vi "均衡解析.vi"(8 "位置":i32, 9 "均衡标记":i32[][](array[numeric]), 11 "均衡引用":refnum<vi>) -> (0 "故障":string[](array[string]), 3 "均衡颜色":u32[](array[colorbox]))   [LabVIEW 2013]
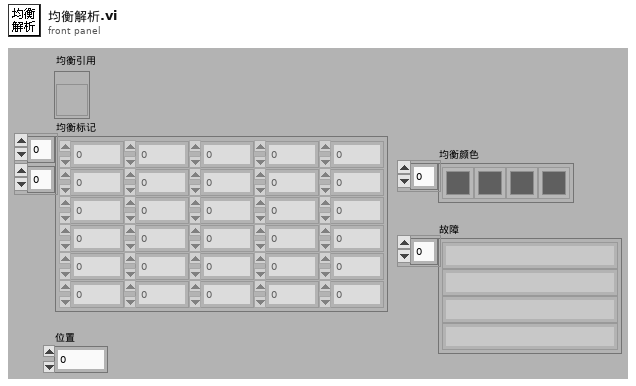
[diagram p1: front panel]
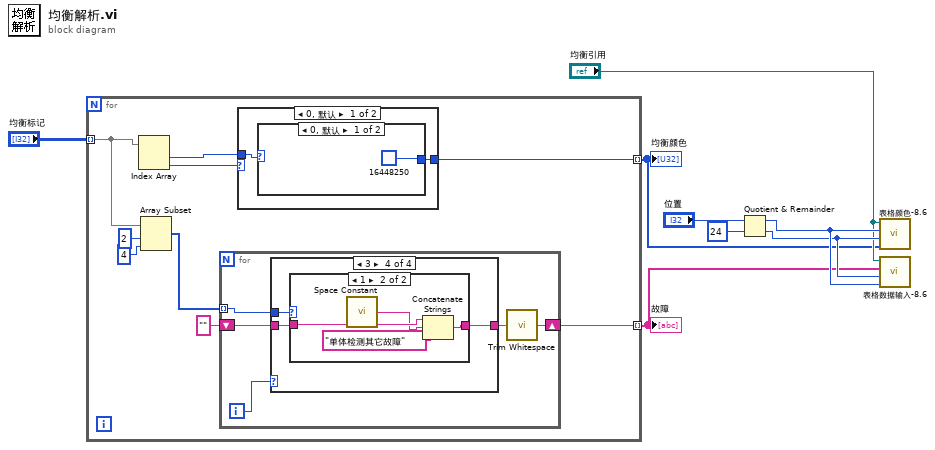
[diagram p0: block diagram]
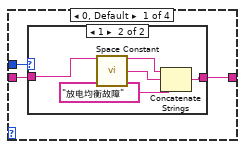
[diagram p2: hidden frame]
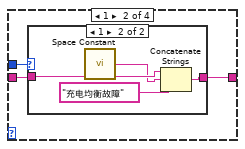
[diagram p4: hidden frame]
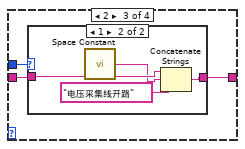
[diagram p6: hidden frame]
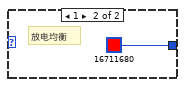
[diagram p9: hidden frame]
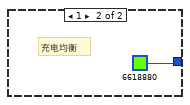
[diagram p10: hidden frame]
diagram:
  n1 = for {
    tunnel: "均衡标记" -> [w14] mode=indexing
    tunnel: [w15] -> w1 mode=indexing
    tunnel: [w9] -> w2 mode=indexing
    n2 = Index Array(array=w14) -> (element #1=w16:i32, element #2=w17:i32)  [unwired: 2 in]
    n3 = Array Subset(array=w14, index=2 ("索引"), length=4 ("长度")) -> (w11:i32[])
    n4 = for {
      tunnel: w11 -> [w22] mode=indexing
      shift-right: [w18] -> w9
      shift-left: "" -> [w20]
      i -> [w19]
      n5 = case shown="3" w19 {
        tunnel: w22 -> [w25 w33 w41 w49]
        tunnel: [w24 w32 w40 w48] -> w21
        tunnel: w20 -> [w23 w31 w39 w47]
        frame 0, Default {
          n6 = case shown="1" w25 {
            tunnel: w23 -> [w26 w28]
            tunnel: [w26 w29] -> w24
            frame 0, Default {
            }
            frame 1 {
              n7 = call <vilib>:"Space Constant.vi"() -> ("String"=w27:string)
              n8 = Concatenate Strings(w28, w27, "放电均衡故障") -> (w29:string)
            }
          }
        }
        frame 1 {
          n9 = case shown="1" w33 {
            tunnel: w31 -> [w34 w36]
            tunnel: [w34 w37] -> w32
            frame 0, Default {
            }
            frame 1 {
              n10 = call <vilib>:"Space Constant.vi"() -> ("String"=w35:string)
              n11 = Concatenate Strings(w36, w35, "充电均衡故障") -> (w37:string)
            }
          }
        }
        frame 2 {
          n12 = case shown="1" w41 {
            tunnel: w39 -> [w42 w44]
            tunnel: [w42 w45] -> w40
            frame 0, Default {
            }
            frame 1 {
              n13 = call <vilib>:"Space Constant.vi"() -> ("String"=w43:string)
              n14 = Concatenate Strings(w44, w43, "电压采集线开路") -> (w45:string)
            }
          }
        }
        frame 3 {
          n15 = case shown="1" w49 {
            tunnel: w47 -> [w50 w52]
            tunnel: [w50 w53] -> w48
            frame 0, Default {
            }
            frame 1 {
              n16 = call <vilib>:"Space Constant.vi"() -> ("String"=w51:string)
              n17 = Concatenate Strings(w52, w51, "单体检测其它故障") -> (w53:string)
            }
          }
        }
      }
      n18 = call <vilib>:"Trim Whitespace.vi"("string"=w21) -> ("trimmed string"=w18:string)  [unwired: 1 in]
    }
    n19 = case shown="0, 默认" w17 {
      tunnel: w16 -> [w56 _]
      tunnel: [w55 u32 6618880] -> w15
      frame 0, Default {
        n20 = case shown="0, 默认" w56 {
          tunnel: [u32 16448250 u32 16711680] -> w55
          frame 0, Default {
          }
          frame 1 {
            # "放电均衡"
          }
        }
      }
      frame 1 {
        # "充电均衡"
      }
    }
  }
  "均衡颜色" <- w1
  "故障" <- w2
  n21 = Quotient & Remainder(x="位置", y=24) -> (x-y*floor(x/y)=w5:i32, floor(x/y)=w4:i32)
  n22 = call "表格颜色-8.6.vi"("颜色类型"=w1, "列数"=w4, "行数"=w5, "表格引用"="均衡引用") -> ()  [unwired: 1 in, 7 out]
  n23 = call "表格数据输入-8.6.vi"("行数"=w5, "列数"=w4, "字符串数组"=w2, "表格引用"="均衡引用") -> ()  [unwired: 8 out]
